vi "Get Number of Channels.vi"(8 "error in":errorcluster, 10 "Group Name":string, 11 "TDMS in":refnum<class "TDMS.lvclass">) -> (0 "error out":errorcluster, 2 "number of channels":i32, 3 "TDMS out":refnum<class "TDMS.lvclass">)   [LabVIEW 2011, in "TDMS.lvclass"]
uses:
  TDMS.lvclass
  TDMS.lvclass/TDMS.ctl
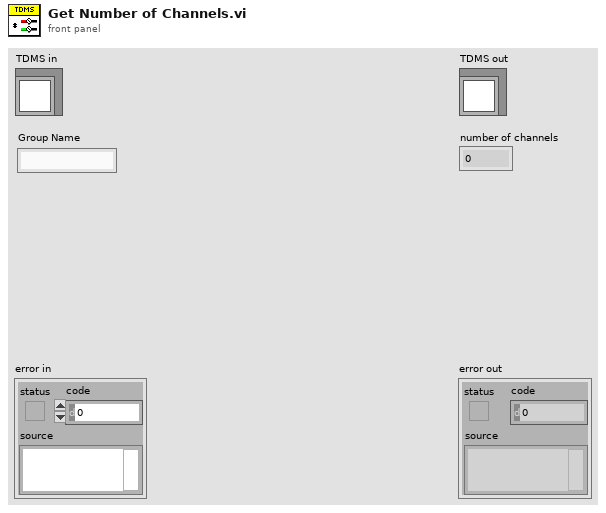
[diagram p1: front panel]
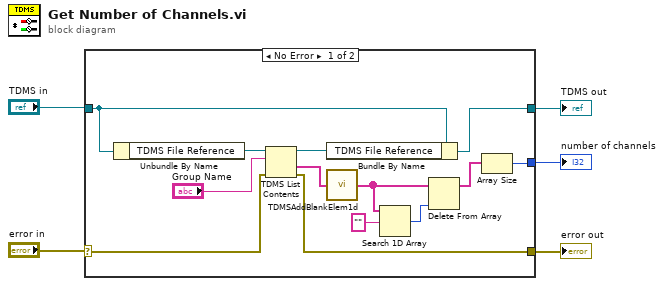
[diagram p0: block diagram]
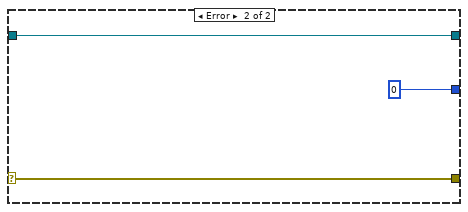
[diagram p2: hidden frame]
diagram:
  n1 = case shown="No Error" "error in" {
    selector: "error in" -> [w11 w21]
    tunnel: [w6 w21] -> w4
    tunnel: [w8 w20] -> w2
    tunnel: "TDMS in" -> [w10 w20]
    tunnel: [w7 0] -> w1
    frame No Error {
      n2 = Unbundle By Name(w10) -> ("TDMS File Reference"=w13:refnum<k34>)
      n3 = TDMS List Contents(4:w11, 6:"Group Name", 7:w13) -> (0:w6:errorcluster, 1:w18:string[], 3:w9:refnum<k34>)  [unwired: 1 out]
      n4 = Bundle By Name(cluster=w10, "TDMS File Reference"=w9) -> (w8:refnum<class "TDMS.lvclass">)
      n5 = call <vilib>:"TDMSAddBlankElem1d.vi"("input string array"=w18) -> ("output string array with blank element at the beginning"=w15:string[])
      n6 = Search 1D Array(1D array=w15, element="") -> (index of element=w17:i32)  [unwired: 1 in]
      n7 = Delete From Array(array=w15, index=w17) -> (array with subset deleted=w14:string[])  [unwired: 1 in, 1 out]
      n8 = Array Size(array=w14) -> (size(s)=w7:i32)
    }
    frame Error {
    }
  }
  "error out" <- w4
  "TDMS out" <- w2
  "number of channels" <- w1
